vi "Example_blinky.vi"() -> ()   [LabVIEW 2022 SP3]
uses:
  usbtmc_scpi_labtool.lvlib
panel:
  out "pin":dbl format="%#_1g"
  out "toggle":bool
  in  "stop":bool
  in  "VISA resource name in":refnum<visa-resource-name>="USB0::0xCAFE::0x4000::123456::INSTR"
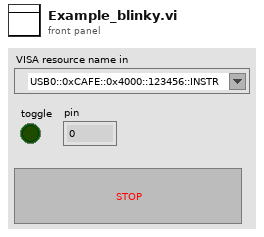
[diagram p1: front panel]
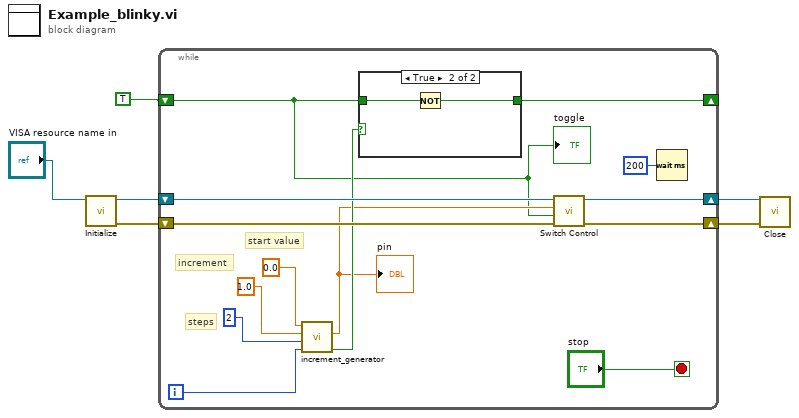
[diagram p0: block diagram]
diagram:
  n1 = call "Initialize.vi"("VISA resource name in"="VISA resource name in") -> ("error out"=w4:errorcluster, "VISA resource name out"=w6:refnum<visa-resource-name>)  [unwired: 9 in]
  n2 = while {
    shift-right: [w20] -> w5
    shift-left: w6 -> [w15]
    shift-right: [w19] -> w3
    shift-left: w4 -> [w14]
    shift-right: [w12] -> _
    shift-left: TRUE -> [w7]
    i -> [w10]
    stop <- "stop" stop-if-true
    # "steps"
    # "increment"
    # "start value"
    n3 = call "increment_generator.vi"("Counter"=w10, "Steps"=u32 2, "Value Increase Per Step"=1.0, "Start Value"=0.0) -> ("Finished"=w11:bool, "Calculated"=w9:dbl)  [unwired: 6 in]
    "pin" <- w9
    n4 = case shown="True" w11 {
      tunnel: w7 -> [w21 w23]
      tunnel: [w21 w22] -> w12
      frame False {
      }
      frame True {
        n5 = Not(x=w23) -> (.not. x?=w22:bool)
      }
    }
    n6 = call "Switch Control.vi"("VISA resource name"=w15, "Pin"=w9, "Enable Input Terminal (F: Off)"=w7, "error in (no error)"=w14) -> ("VISA resource name out"=w20:refnum<visa-resource-name>, "error out"=w19:errorcluster)  [unwired: 5 in]
    n7 = Wait (ms)(milliseconds to wait=u32 200) -> ()  [unwired: 1 out]
    "toggle" <- w7
  }
  n8 = call "Close.vi"("error in (no error)"=w3, "VISA resource name"=w5) -> ()  [unwired: 10 in]
